vi "IMAQMemory.vi"() -> (1 "Bytes in use":u64, 2 "Images in use":i32)   [LabVIEW 2011]
uses:
  NIVision.dll
panel:
  # "check / estimate used IMAQ space"
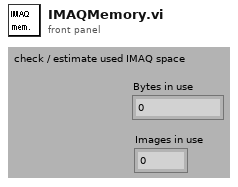
[diagram p1: front panel]
types:
  T1 = enum16{"status", "createIMAQ", "getIMAQ", "getNumber", "deleteIMAQ", "deleteAll", "MemoryUsage", "GetAccess", "DecreaseAccess", "ActualIndex", "ElementToNumber"}
  T2 = cluster{"Start":u32, "Length":u32, "Image Type":enum32{"8 bits", "16 bits", "Float", "Complex", "RGB Chunky"}, "Width":u32, "Height":u32, "Size":u32}[]
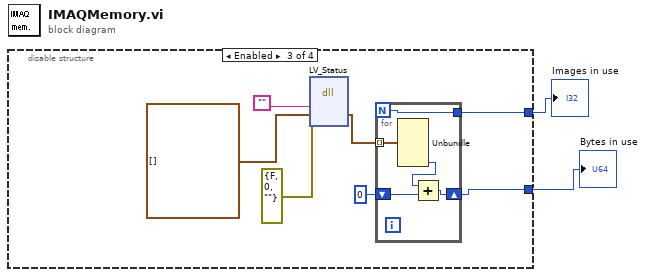
[diagram p0: block diagram]
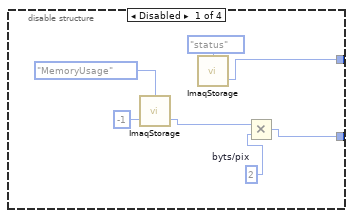
[diagram p2: hidden frame]
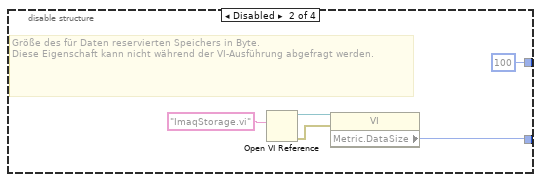
[diagram p3: hidden frame]
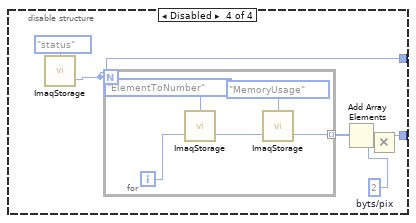
[diagram p4: hidden frame]
diagram:
  n1 = disable-structure shown="Enabled" {
    disable-tunnel: [w5 w13 w15 w29] -> w2
    disable-tunnel: [w3 100 ("Images in use") w17 w27] -> w1
    frame Disabled {
      w6 = u64 2  # byts/pix
      n2 = call "ImaqStorage.vi"("Number"=-1, "Command"=T1."MemoryUsage") -> ("Number out"=w7:i32)  [unwired: 1 in, 1 out]
      n3 = call "ImaqStorage.vi"("Command"=T1."status") -> ("Number out"=w3:i32)  [unwired: 2 in, 1 out]
      n4 = Multiply(x=w7, y=w6) -> (x*y=w5:u64)
    }
    frame Disabled {
      # "Größe des für Daten reservierten Speichers in Byte. \nDiese Eigenschaft kann nicht während der VI-Ausführung abgefragt werden."
      n5 = Open VI Reference(vi path="ImaqStorage.vi") -> (vi reference=w14:refnum<vi>, error out=w11:errorcluster)  [unwired: 5 in]
      n6 = property class="VI"(reference=w14, error in=w11) -> ("Metric.DataSize"=w13:u32)  [unwired: 2 out]
    }
    frame Enabled {
      n7 = dll-call lib="NIVision.dll" fn="LV_Status"("allNames"="", T2 [], "error in (no error)"=errorcluster {"status"=FALSE, "code"=0, "source"=""}) -> (w18:T2)  [unwired: 6 in, 2 out]
      n8 = for {
        N -> [w25]
        tunnel: w18 -> [w26] mode=indexing
        tunnel: [w25] -> w17
        shift-right: [w22] -> w15
        shift-left: u64 0 -> [w23]
        n9 = Unbundle(w26) -> ("Size"=w24:u32)  [unwired: 5 out]
        n10 = Add(x=w24, y=w23) -> (x+y=w22:u64)
      }
    }
    frame Disabled {
      w28 = u64 2  # byts/pix
      n11 = call "ImaqStorage.vi"("Command"=T1."status") -> ("Number out"=w27:i32)  [unwired: 2 in, 1 out]
      n12 = for {
        N: w27 -> [_]
        tunnel: [w33] -> w31 mode=indexing
        i -> [w36]
        n13 = call "ImaqStorage.vi"("Number"=w36, "Command"=T1."ElementToNumber") -> ("Number out"=w35:i32)  [unwired: 1 in, 1 out]
        n14 = call "ImaqStorage.vi"("Number"=w35, "Command"=T1."MemoryUsage") -> ("Number out"=w33:i32)  [unwired: 1 in, 1 out]
      }
      n15 = Add Array Elements(numeric array=w31) -> (sum=w30:i32)
      n16 = Multiply(x=w30, y=w28) -> (x*y=w29:u64)
    }
  }
  "Bytes in use" <- w2
  "Images in use" <- w1
